vi "Initialize.vi"(8 "error in (no error)":errorcluster, 9 "Reset (True)":bool=TRUE, 10 "ID Query (True)":bool=TRUE, 11 "VISA resource name":refnum<visa-resource-name>) -> (0 "error out":errorcluster, 2 "idn string":string, 3 "VISA resource name out":refnum<visa-resource-name>)   [LabVIEW 2020, in "Agilent 3458.lvlib"]
doc: "Establishes communication with the instrument and optionally performs an instrument identification query and/or an instrument reset. It also places the instrument in a default state needed for other instrument driver operations. Therefore, call this VI before calling other instrument driver VIs for this instrument. Generally, you need to call the Initialize VI only once at the beginning of an application."
uses:
  Agilent 3458.lvlib
panel:
  # "(c) 2007  National Instruments.  ALL RIGHTS RESERVED."
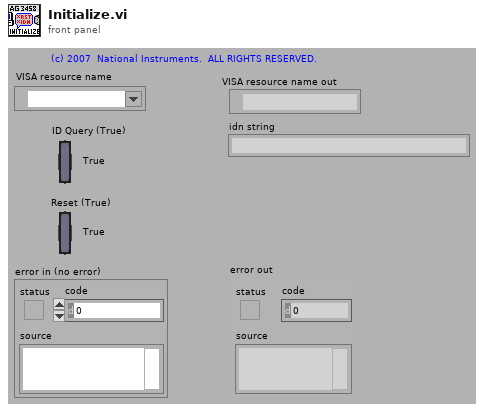
[diagram p1: front panel]
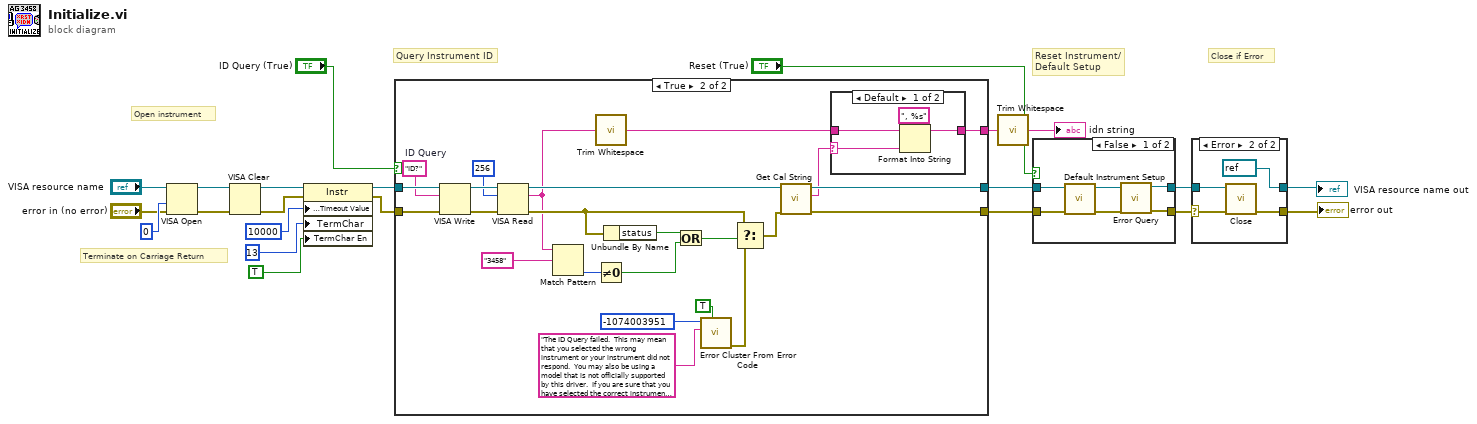
[diagram p0: block diagram]
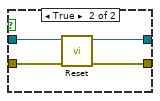
[diagram p3: hidden frame]
diagram:
  # "Terminate on Carriage Return"
  # "Close if Error"
  # "Query Instrument ID"
  # "Reset Instrument/\nDefault Setup"
  # "Open instrument"
  n1 = VISA Open(access mode=u32 0, error in (no error)="error in (no error)", VISA resource name="VISA resource name") -> (VISA resource name=w15:refnum<visa-resource-name>, error out=w14:errorcluster)  [unwired: 2 in]
  n2 = VISA Clear(VISA resource name=w15, error in (no error)=w14) -> (VISA resource name out=w13:refnum<visa-resource-name>, error out=w12:errorcluster)
  n3 = property class="Instr"(reference=w13, error in=w12, "General Settings:Timeout Value"=u32 10000, "TermChar"=u8 13 ("Message Based Settings:Termination Character"), "TermChar En"=TRUE ("Message Based Settings:Termination Character Enable")) -> (reference out=w18:refnum<visa-resource-name>, error out=w17:errorcluster)
  n4 = case shown="True" "ID Query (True)" {
    tunnel: [w23 w32] -> w21
    tunnel: [w24 w31] -> w22
    tunnel: w18 -> [w24 w47]
    tunnel: w17 -> [w23 w48]
    tunnel: [_ w25] -> w2
    frame False {
    }
    frame True {
      w42 = "ID?"  # ID Query
      n5 = VISA Write(VISA resource name=w47, write buffer=w42, error in (no error)=w48) -> (VISA resource name out=w46:refnum<visa-resource-name>, error out=w45:errorcluster)  [unwired: 1 out]
      n6 = VISA Read(VISA resource name=w46, byte count=u32 256, error in (no error)=w45) -> (VISA resource name out=w30:refnum<visa-resource-name>, read buffer=w28:string, error out=w33:errorcluster)  [unwired: 1 out]
      n7 = Match Pattern(string=w28, regular expression="3458") -> (offset past match=w37:i32)  [unwired: 1 in, 3 out]
      n8 = call <vilib>:"Trim Whitespace.vi"("string"=w28) -> ("trimmed string"=w26:string)  [unwired: 1 in]
      n9 = Not Equal To 0?(x=w37) -> (x != 0?=w34:bool)
      n10 = Unbundle By Name(w33) -> ("status"=w36:bool)
      n11 = Or(x=w36, y=w34) -> (x .or. y?=w35:bool)
      n12 = call <vilib>:"Error Cluster From Error Code.vi"("show call chain? (False)"=TRUE, "error message (\"\")"="The ID Query failed.  This may mean that you selected the wrong instrument or your instrument did not respond.  You may also be using a model that is not officially supported by this driver.  If you are sure that you have selected the correct instrument and it is responding, try disabling the ID Query." ("Source (VI Name)"), "error code (0)"=-1074003951 ("Code")) -> ("error out"=w41:errorcluster)  [unwired: 6 in]
      n13 = Select(t=w33, s=w35, f=w41) -> (s? t:f=w29:errorcluster)
      n14 = call "Get Cal String.vi"("error in(no error)"=w29, "VISA Resource Name"=w30) -> ("error out"=w32:errorcluster, "calibration string"=w27:string, "VISA resource name out"=w31:refnum<visa-resource-name>)  [unwired: 7 in]
      n15 = case shown="Default" w27 {
        selector: w27 -> [w50 _]
        tunnel: [w49 w53] -> w25
        tunnel: w26 -> [w52 w53]
        frame Default {
          n16 = Format Into String(format string=", %s", initial string=w52, w50) -> (resulting string=w49:string)  [unwired: 1 in, 1 out]
        }
        frame "" {
        }
      }
    }
  }
  n17 = call <vilib>:"Trim Whitespace.vi"("string"=w2) -> ("trimmed string"=→"idn string":string)  [unwired: 1 in]
  n18 = case shown="False" "Reset (True)" {
    tunnel: w21 -> [w58 w61]
    tunnel: [w54 w60] -> w10
    tunnel: w22 -> [w59 w62]
    tunnel: [w55 w63] -> w11
    frame False {
      n19 = call "Default Instrument Setup.vi"("error in (no error)"=w58, "VISA resource name"=w59) -> ("error out"=w56:errorcluster, "VISA resource name out"=w57:refnum<visa-resource-name>)  [unwired: 8 in]
      n20 = call "Error Query.vi"("error in (no error)"=w56, "VISA resource name"=w57) -> ("error out"=w54:errorcluster, "VISA resource name out"=w55:refnum<visa-resource-name>)  [unwired: 6 in, 2 out]
    }
    frame True {
      n21 = call "Reset.vi"("error in (no error)"=w61, "VISA resource name"=w62) -> ("error out"=w60:errorcluster, "VISA resource name out"=w63:refnum<visa-resource-name>)  [unwired: 8 in]
    }
  }
  n22 = case shown="Error" w10 {
    selector: w10 -> [w64 w67]
    tunnel: w11 -> [w65 w68]
    tunnel: [w65 refnum<visa-resource-name> refnum ("VISA resource name out")] -> w5
    tunnel: [w64 w69] -> w3
    frame No Error {
    }
    frame Error {
      n23 = call "Close.vi"("error in (no error)"=w67, "VISA resource name"=w68) -> ("error out"=w69:errorcluster)  [unwired: 9 in]
    }
  }
  "VISA resource name out" <- w5
  "error out" <- w3
